vi "Run Filter.vi"(8 "错误输入（无错误）":errorcluster caption="Error In(No Error)", 11 "CAN Device In":T1={"Device Type"=20, "Device Index"=0, "CANInd"=0, "Baud(E_U)"=1835016} {"Baud(E_U)" items=["1000Kbps"=393219, "800Kbps"=393220, "500Kbps"=393223, "250Kbps"=1835016, "125Kbps"=1835025, "100Kbps"=1441827, "50Kbps"=1835052, "20Kbps"=1441971, "10Kbps"=1835232, "5Kbps"=1835457]; "Device Type" items=["PCI5121"=1, "PCI9810"=2, "USBCAN1"=3, "USBCAN2"=4, "PCI9820"=5, "PCI5110"=7, "PC104CAN"=11, "CANETUDP"=12, "PCI9840B"=14, "PC104C2"=15, "PCI9820I"=16, "CANETTCP"=17, "PCIE9221"=24, "PCI5010U"=19, "USBCAN_E_U"=20, "USBCAN_2E_U"=21, "PCI5020U"=22, "PCIE9120I"=27, "PCIE9110I"=28, "PCIE9140I"=29, "USBCAN-4E-U"=31, "USBCAN-8E-U"=34]}) -> (0 "错误输出":errorcluster caption="Error Out", 3 "CAN Device Out":T1={"Device Type"=20, "Device Index"=0, "CANInd"=0, "Baud(E_U)"=1835016} {"Baud(E_U)" items=["1000Kbps"=393219, "800Kbps"=393220, "500Kbps"=393223, "250Kbps"=1835016, "125Kbps"=1835025, "100Kbps"=1441827, "50Kbps"=1835052, "20Kbps"=1441971, "10Kbps"=1835232, "5Kbps"=1835457]; "Device Type" items=["PCI5121"=1, "PCI9810"=2, "USBCAN1"=3, "USBCAN2"=4, "PCI9820"=5, "PCI5110"=7, "PC104CAN"=11, "CANETUDP"=12, "PCI9840B"=14, "PC104C2"=15, "PCI9820I"=16, "CANETTCP"=17, "PCIE9221"=24, "PCI5010U"=19, "USBCAN_E_U"=20, "USBCAN_2E_U"=21, "PCI5020U"=22, "PCIE9120I"=27, "PCIE9110I"=28, "PCIE9140I"=29, "USBCAN-4E-U"=31, "USBCAN-8E-U"=34]})   [LabVIEW 2020, in "ZLGCAN.lvclass"]
uses:
  ZLGCAN.lvclass
  Device.ctl
  ControlCAN.dll
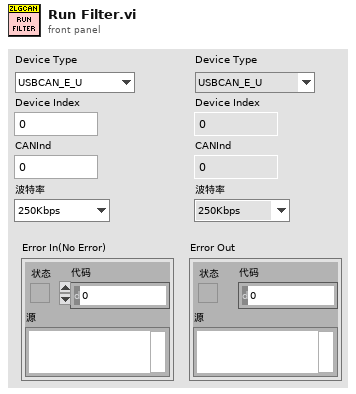
[diagram p1: front panel]
types:
  T1 = typedef "ZLGCAN.lvclass/Device.ctl" = cluster{"Device Type":u32, "Device Index":u32, "CANInd":u32, "Baud(E_U)":u32}
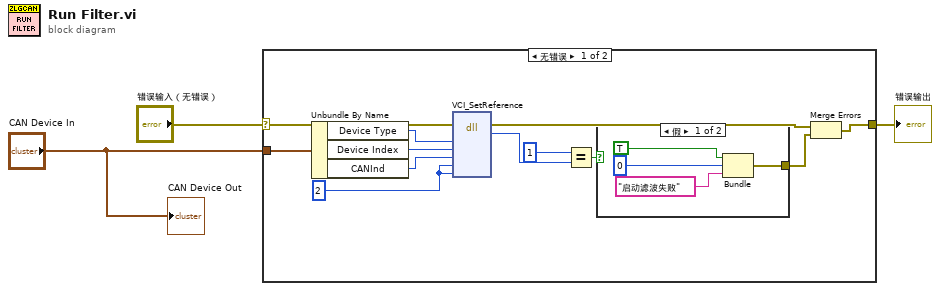
[diagram p0: block diagram]
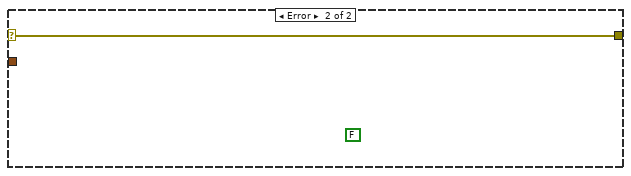
[diagram p3: hidden frame]
diagram:
  n1 = case shown="无错误" "错误输入（无错误）" {
    selector: "错误输入（无错误）" -> [w5 w20]
    tunnel: [w14 w20] -> w2
    tunnel: "CAN Device In" -> [w4 _]
    frame No Error {
      w6 = u32 2 ("RefType")
      n2 = Unbundle By Name(w4) -> ("Device Type"=w9:u32, "Device Index"=w8:u32, "CANInd"=w7:u32)
      n3 = dll-call lib="PTH2sabs CUsersxu.dongDesktop新建文件夹新建文件夹 (2) - 副本ZLGCAN\nControlCANControlCAN.dll" fn="VCI_SetReference"(error in=w5, "DevType"=w9, "DevIndex"=w8, "CANInd"=w7, "RefType"=w6, "pData"=w6) -> (error out=w11:errorcluster, "返回类型"=w12:u32)  [unwired: 7 in, 1 out]
      n4 = Equal?(x=u32 1 ("y"), y=w12) -> (x = y?=w10:bool)
      n5 = case shown="假" w10 {
        tunnel: [w16 _] -> w15
        frame False {
          n6 = Bundle("status"=TRUE, "code"=0, "消息"="启动滤波失败") -> (w16:cluster{"status":bool, "code":i32, "消息":string})  [unwired: 1 in]
        }
        frame True {
        }
      }
      n7 = Merge Errors(w11, w15) -> (w14:errorcluster)
    }
    frame Error {
      (unwired) FALSE
    }
  }
  "错误输出" <- w2
  "CAN Device Out" <- "CAN Device In"
